vi "(Un)Lock FrontPanel.vi"(9 "SetDeferPanel?":bool=TRUE, 10 "Lock?":bool=TRUE, 11 "Tree Reference":refnum<vi>) -> ()   [LabVIEW 2014, in "CS++MessageMakerMain.lvlib" / "CS++MessageMakerMain.lvclass"]
uses:
  CS++MessageMakerMain.lvclass
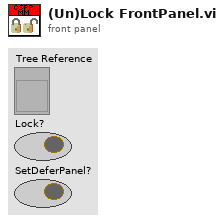
[diagram p1: front panel]
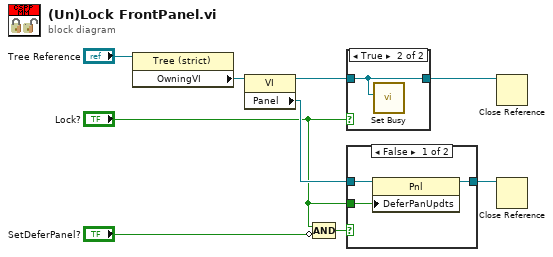
[diagram p0: block diagram]
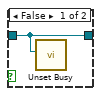
[diagram p3: hidden frame]
diagram:
  n1 = property class="Tree (strict)"(reference="Tree Reference") -> ("OwningVI"=w9:refnum<vi>)  [unwired: 1 in, 2 out]
  n2 = property class="VI"(reference=w9) -> (reference out=w7:refnum<vi>, "Panel"=w4:refnum<vi>)  [unwired: 1 in, 1 out]
  n3 = Compound Arithmetic op=AND("Lock?", invert "SetDeferPanel?") -> (w3:bool)
  n4 = case shown="True" "Lock?" {
    tunnel: w7 -> [w10 w11]
    tunnel: [w10 w11] -> w6
    frame False {
      n5 = call <vilib>:"Unset Busy.vi"("VI reference (current VI)"=w10) -> ()  [unwired: 10 in, 1 out]
    }
    frame True {
      n6 = call <vilib>:"Set Busy.vi"("VI reference (current VI)"=w11) -> ()  [unwired: 9 in, 2 out]
    }
  }
  n7 = case shown="False" w3 {
    tunnel: w4 -> [w14 w15]
    tunnel: [w13 w15] -> w8
    tunnel: "Lock?" -> [w12 _]
    frame False {
      n8 = property class="Pnl"(reference=w14, "DeferPanUpdts"=w12) -> (reference out=w13:refnum<vi>)  [unwired: 1 in, 1 out]
    }
    frame True {
    }
  }
  n9 = Close Reference(reference=w6) -> ()  [unwired: 1 in, 1 out]
  n10 = Close Reference(reference=w8) -> ()  [unwired: 1 in, 1 out]
